vi "Save GUI Settings (SubVI).vi"(8 "Settings File Name":path=path "C:/MWT/Config.ini", 11 "GUI Parameters":T1={"Image Width"=3072, "Image Height"=3072, "Pixel Intensity Low"=25, "Pixel Intensity High"=135, "Box Side Low"=6, "Box Side High"=200, "Box W+L Low"=12, "Box W+L High"=200, "Area Low"=12, "Area High"=200, "BG SUB TH"=200, "N Spine Points"=11.0, "Min Contour Points"=200, "Pixel Resolution (um/Pixel)"=40.69, "Gamma"=0.2} {"Gamma" format="%#_13g"; "Pixel Resolution (um/Pixel)" format="%#_13g"}) -> ()   [LabVIEW 2020]
uses:
  Controls (HOST)/GUI Param.ctl
  Controls (HOST)/GUI Param List.ctl
  <vilib>/Utility/config.llb/Write Key (U32).vi
  <vilib>/Utility/config.llb/Write Key (I32).vi
  <vilib>/Utility/config.llb/Write Key (Double).vi
  <vilib>/Utility/config.llb/NI_LVConfig.lvlib
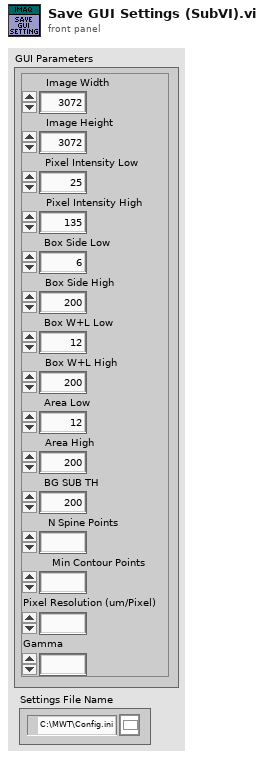
[diagram p1: front panel]
types:
  T1 = typedef "GUI Param.ctl" = cluster{"Image Width":u16, "Image Height":u16, "Pixel Intensity Low":u8, "Pixel Intensity High":u8, "Box Side Low":u32, "Box Side High":u32, "Box W+L Low":u32, "Box W+L High":u32, "Area Low":u32, "Area High":u32, "BG SUB TH":i16, "N Spine Points":fxp<+,8,8>, "Min Contour Points":u16, "Pixel Resolution (um/Pixel)":dbl, "Gamma":dbl}
  T2 = typedef "GUI Param List.ctl" = enum16{"None", "Image Height", "Image Width", "Pixel Intensity Low", "Pixel Intensity High", "Box Side Low", "Box Side High", "Box W+L Low", "Box W+L High", "Area Low", "Area High", "BG Sub Threshold", "N Spine Points", "Min Contour Points", "Pixel Resolution", "Gamma"}
  T3 = typedef "NI_LVConfig.lvlib/Config Data RefNum.ctl" = refnum<k1>
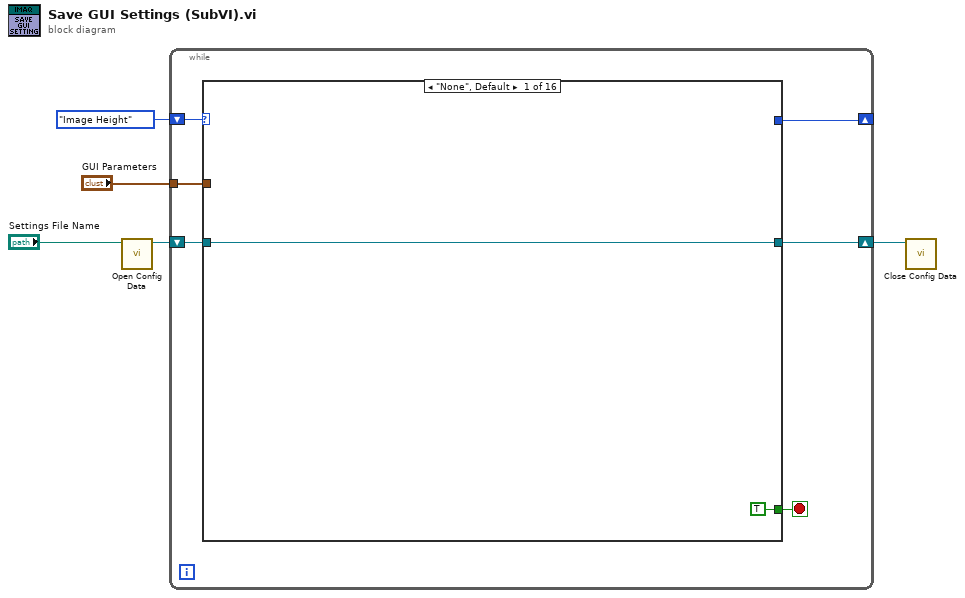
[diagram p0: block diagram]
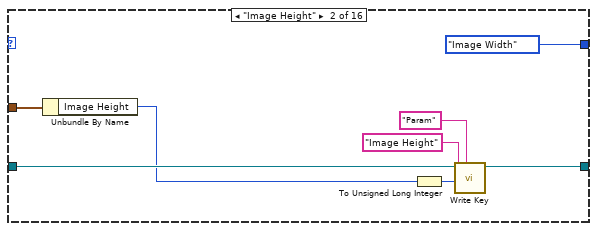
[diagram p2: hidden frame]
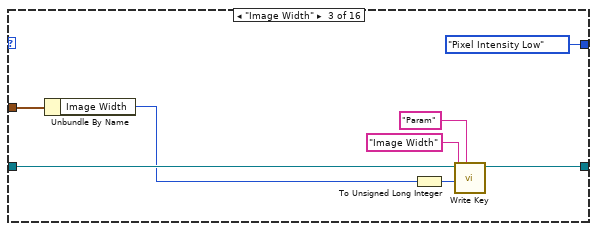
[diagram p3: hidden frame]
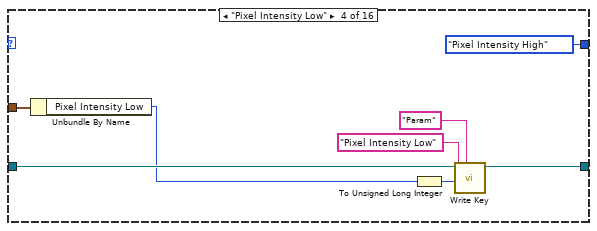
[diagram p4: hidden frame]
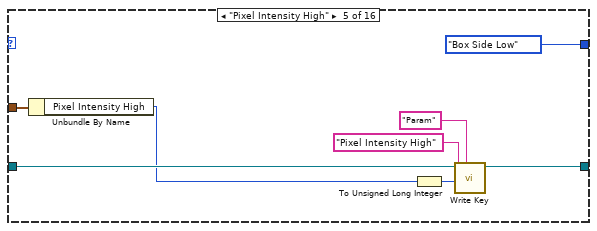
[diagram p5: hidden frame]
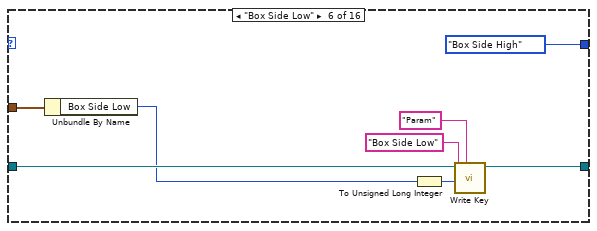
[diagram p6: hidden frame]
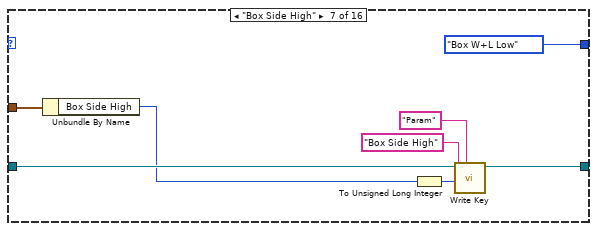
[diagram p7: hidden frame]
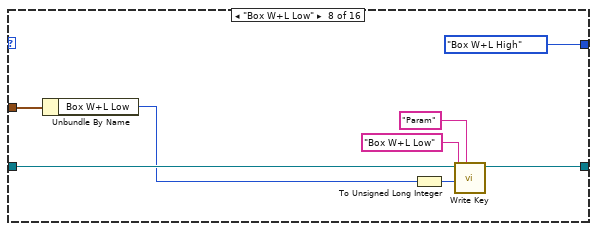
[diagram p8: hidden frame]
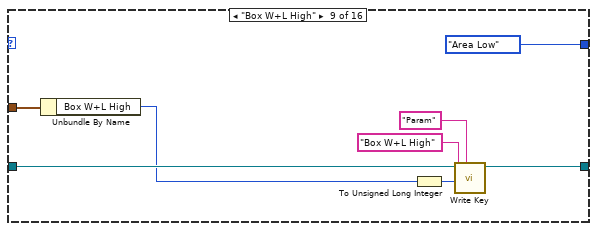
[diagram p9: hidden frame]
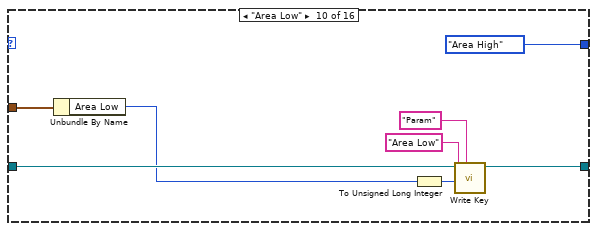
[diagram p10: hidden frame]
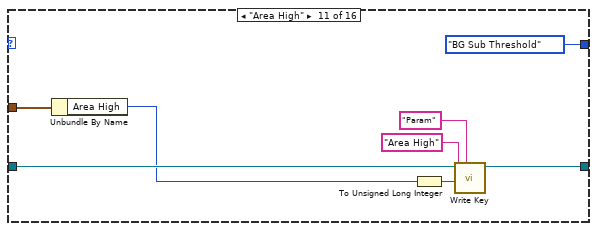
[diagram p11: hidden frame]
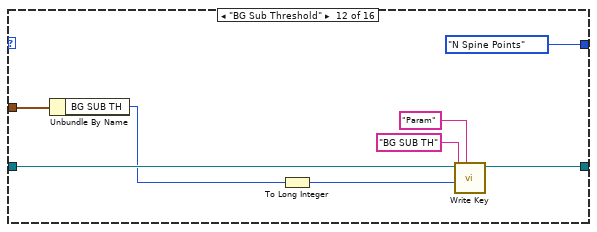
[diagram p12: hidden frame]
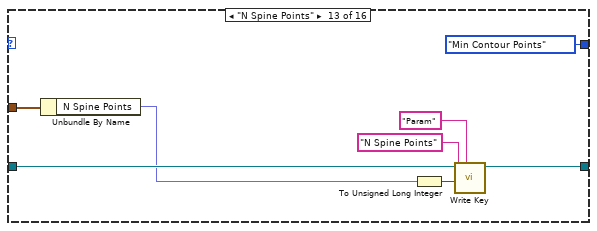
[diagram p13: hidden frame]
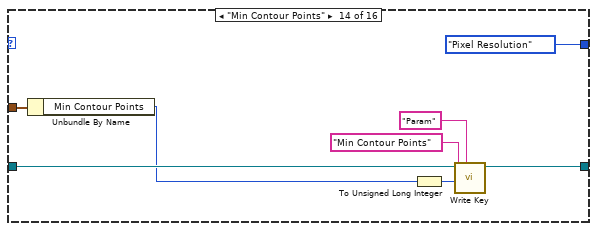
[diagram p14: hidden frame]
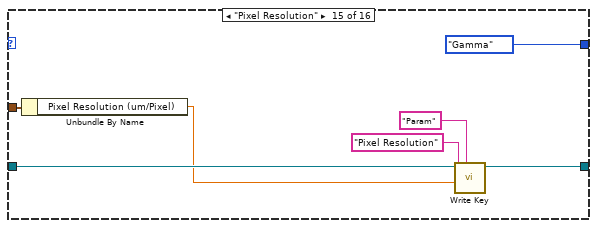
[diagram p15: hidden frame]
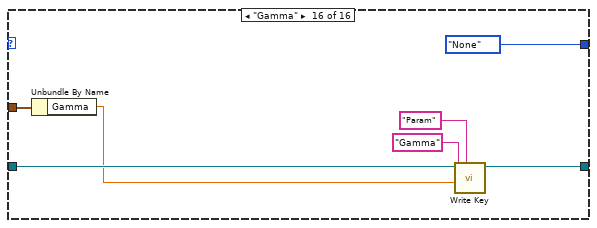
[diagram p16: hidden frame]
diagram:
  n1 = call <vilib>:"Open Config Data.vi"("configuration file path"="Settings File Name") -> ("refnum"=w5:T3)  [unwired: 8 in, 2 out]
  n2 = while {
    shift-right: [w10] -> w3
    shift-left: w5 -> [w11]
    shift-right: [w7] -> _
    shift-left: GUI_Param_List."Image Height" -> [w9]
    tunnel: "GUI Parameters" -> [w6]
    stop <- w8 stop-if-true
    n3 = case shown="\"None\", Default" w9 {
      tunnel: w11 -> [w13 w21 w29 w37 w45 w53 w61 w69 w77 w85 w93 w101 w109 w117 w124 w131]
      tunnel: [w13 w20 w28 w36 w44 w52 w60 w68 w76 w84 w92 w100 w108 w116 w123 w130] -> w10
      tunnel: [TRUE _ _ _ _ _ _ _ _ _ _ _ _ _ _ _] -> w8
      tunnel: [_ GUI_Param_List."Image Width" GUI_Param_List."Pixel Intensity Low" GUI_Param_List."Pixel Intensity High" GUI_Param_List."Box Side Low" GUI_Param_List."Box Side High" GUI_Param_List."Box W+L Low" GUI_Param_List."Box W+L High" GUI_Param_List."Area Low" GUI_Param_List."Area High" GUI_Param_List."BG Sub Threshold" GUI_Param_List."N Spine Points" GUI_Param_List."Min Contour Points" GUI_Param_List."Pixel Resolution" GUI_Param_List."Gamma" GUI_Param_List."None"] -> w7
      tunnel: w6 -> [_ w18 w26 w34 w42 w50 w58 w66 w74 w82 w90 w98 w106 w114 w121 w128]
      frame "None", Default {
      }
      frame "Image Height" {
        n4 = Unbundle By Name(w18) -> ("Image Height"=w17:u16)
        n5 = To Unsigned Long Integer(number=w17) -> (unsigned 32bit integer=w15:u32)
        n6 = call-poly <vilib>:"Write Key.vi"("section"="Param", "value"=w15, "key"="Image Height" ("section"), "refnum"=w21) -> ("refnum out"=w20:T3)  [unwired: 5 in, 2 out]
      }
      frame "Image Width" {
        n7 = Unbundle By Name(w26) -> ("Image Width"=w25:u16)
        n8 = To Unsigned Long Integer(number=w25) -> (unsigned 32bit integer=w23:u32)
        n9 = call-poly <vilib>:"Write Key.vi"("section"="Param", "value"=w23, "key"="Image Width" ("section"), "refnum"=w29) -> ("refnum out"=w28:T3)  [unwired: 5 in, 2 out]
      }
      frame "Pixel Intensity Low" {
        n10 = Unbundle By Name(w34) -> ("Pixel Intensity Low"=w33:u8)
        n11 = To Unsigned Long Integer(number=w33) -> (unsigned 32bit integer=w31:u32)
        n12 = call-poly <vilib>:"Write Key.vi"("section"="Param", "value"=w31, "key"="Pixel Intensity Low" ("section"), "refnum"=w37) -> ("refnum out"=w36:T3)  [unwired: 5 in, 2 out]
      }
      frame "Pixel Intensity High" {
        n13 = Unbundle By Name(w42) -> ("Pixel Intensity High"=w41:u8)
        n14 = To Unsigned Long Integer(number=w41) -> (unsigned 32bit integer=w39:u32)
        n15 = call-poly <vilib>:"Write Key.vi"("section"="Param", "value"=w39, "key"="Pixel Intensity High" ("section"), "refnum"=w45) -> ("refnum out"=w44:T3)  [unwired: 5 in, 2 out]
      }
      frame "Box Side Low" {
        n16 = Unbundle By Name(w50) -> ("Box Side Low"=w49:u32)
        n17 = To Unsigned Long Integer(number=w49) -> (unsigned 32bit integer=w47:u32)
        n18 = call-poly <vilib>:"Write Key.vi"("section"="Param", "value"=w47, "key"="Box Side Low" ("section"), "refnum"=w53) -> ("refnum out"=w52:T3)  [unwired: 5 in, 2 out]
      }
      frame "Box Side High" {
        n19 = Unbundle By Name(w58) -> ("Box Side High"=w57:u32)
        n20 = To Unsigned Long Integer(number=w57) -> (unsigned 32bit integer=w55:u32)
        n21 = call-poly <vilib>:"Write Key.vi"("section"="Param", "value"=w55, "key"="Box Side High" ("section"), "refnum"=w61) -> ("refnum out"=w60:T3)  [unwired: 5 in, 2 out]
      }
      frame "Box W+L Low" {
        n22 = Unbundle By Name(w66) -> ("Box W+L Low"=w65:u32)
        n23 = To Unsigned Long Integer(number=w65) -> (unsigned 32bit integer=w63:u32)
        n24 = call-poly <vilib>:"Write Key.vi"("section"="Param", "value"=w63, "key"="Box W+L Low" ("section"), "refnum"=w69) -> ("refnum out"=w68:T3)  [unwired: 5 in, 2 out]
      }
      frame "Box W+L High" {
        n25 = Unbundle By Name(w74) -> ("Box W+L High"=w73:u32)
        n26 = To Unsigned Long Integer(number=w73) -> (unsigned 32bit integer=w71:u32)
        n27 = call-poly <vilib>:"Write Key.vi"("section"="Param", "value"=w71, "key"="Box W+L High" ("section"), "refnum"=w77) -> ("refnum out"=w76:T3)  [unwired: 5 in, 2 out]
      }
      frame "Area Low" {
        n28 = Unbundle By Name(w82) -> ("Area Low"=w81:u32)
        n29 = To Unsigned Long Integer(number=w81) -> (unsigned 32bit integer=w79:u32)
        n30 = call-poly <vilib>:"Write Key.vi"("section"="Param", "value"=w79, "key"="Area Low" ("section"), "refnum"=w85) -> ("refnum out"=w84:T3)  [unwired: 5 in, 2 out]
      }
      frame "Area High" {
        n31 = Unbundle By Name(w90) -> ("Area High"=w89:u32)
        n32 = To Unsigned Long Integer(number=w89) -> (unsigned 32bit integer=w87:u32)
        n33 = call-poly <vilib>:"Write Key.vi"("section"="Param", "value"=w87, "key"="Area High" ("section"), "refnum"=w93) -> ("refnum out"=w92:T3)  [unwired: 5 in, 2 out]
      }
      frame "BG Sub Threshold" {
        n34 = Unbundle By Name(w98) -> ("BG SUB TH"=w97:i16)
        n35 = To Long Integer(number=w97) -> (32bit integer=w94:i32)
        n36 = call-poly <vilib>:"Write Key.vi"("section"="Param", "value"=w94, "key"="BG SUB TH" ("section"), "refnum"=w101) -> ("refnum out"=w100:T3)  [unwired: 5 in, 2 out]
      }
      frame "N Spine Points" {
        n37 = Unbundle By Name(w106) -> ("N Spine Points"=w105:fxp<+,8,8>)
        n38 = To Unsigned Long Integer(number=w105) -> (unsigned 32bit integer=w103:u32)
        n39 = call-poly <vilib>:"Write Key.vi"("section"="Param", "value"=w103, "key"="N Spine Points" ("section"), "refnum"=w109) -> ("refnum out"=w108:T3)  [unwired: 5 in, 2 out]
      }
      frame "Min Contour Points" {
        n40 = Unbundle By Name(w114) -> ("Min Contour Points"=w113:u16)
        n41 = To Unsigned Long Integer(number=w113) -> (unsigned 32bit integer=w111:u32)
        n42 = call-poly <vilib>:"Write Key.vi"("section"="Param", "value"=w111, "key"="Min Contour Points" ("section"), "refnum"=w117) -> ("refnum out"=w116:T3)  [unwired: 5 in, 2 out]
      }
      frame "Pixel Resolution" {
        n43 = Unbundle By Name(w121) -> ("Pixel Resolution (um/Pixel)"=w120:dbl)
        n44 = call-poly <vilib>:"Write Key.vi"("section"="Param", "value"=w120, "key"="Pixel Resolution" ("section"), "refnum"=w124) -> ("refnum out"=w123:T3)  [unwired: 5 in, 2 out]
      }
      frame "Gamma" {
        n45 = Unbundle By Name(w128) -> ("Gamma"=w127:dbl)
        n46 = call-poly <vilib>:"Write Key.vi"("section"="Param", "value"=w127, "key"="Gamma" ("section"), "refnum"=w131) -> ("refnum out"=w130:T3)  [unwired: 5 in, 2 out]
      }
    }
  }
  n47 = call <vilib>:"Close Config Data.vi"("refnum"=w3) -> ()  [unwired: 9 in, 2 out]
